vi "layout.vi"(0 "reference":refnum<class "FinalStateNode.lvclass">, 1 "graph":refnum<class "Graph.lvclass">, 2 "graphics":refnum<class "Graphics.lvclass">, 3 "grid":refnum<class "Grid.lvclass">, 5 "error in (no error)":errorcluster) -> (14 "reference out":refnum<class "FinalStateNode.lvclass">, 19 "error out":errorcluster)   [LabVIEW 2012, in "FinalStateNode.lvclass"]
doc: "public void layout(Graph g, Graphics2D g2, Grid grid)"
uses:
  <resource>/Framework/Providers/Open_GDS/UML/FinalStateNode_class/FinalStateNode.lvclass
  <resource>/Framework/Providers/Open_GDS/UML/Graph_class/Graph.lvclass
  <resource>/Framework/Providers/Open_GDS/UML/Graphics_class/Graphics.lvclass
  <resource>/Framework/Providers/Open_GDS/UML/Grid_class/Grid.lvclass
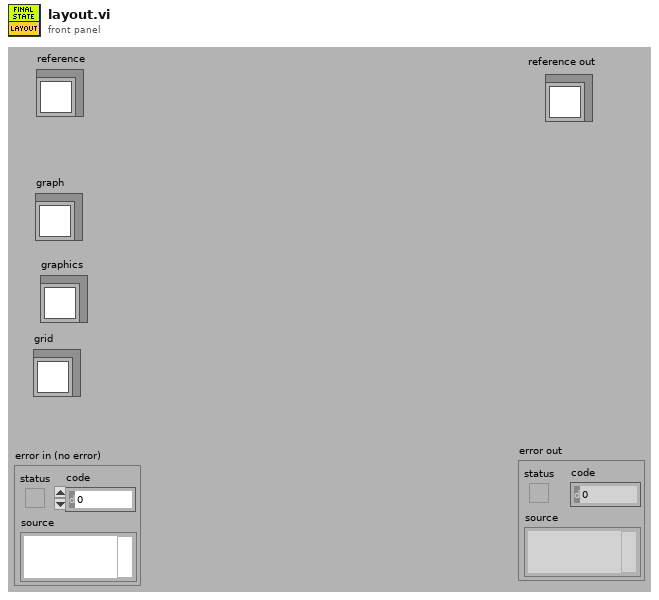
[diagram p1: front panel]
types:
  T1 = typedef "FinalStateNode.lvclass/ObjectAttributes.ctl" = cluster{"Base class":T2, "name":refnum<class "MultiLineString.lvclass">, "DEFAULT_WIDTH":i32, "DEFAULT_HEIGHT":i32}
  T2 = typedef "RectangularNode.lvclass/ObjectAttributes.ctl" = cluster{"Base class":T3, "bounds":T4}
  T3 = typedef "AbstractNode.lvclass/ObjectAttributes.ctl" = cluster{"parent":refnum<class "AbstractNode.lvclass">, "children":refnum<class "AbstractNode.lvclass">[], "Hidden":bool}
  T4 = typedef "Rectangle Rectangle2D.ctl" = cluster{"x":dbl, "y":dbl, "width":dbl, "height":dbl}
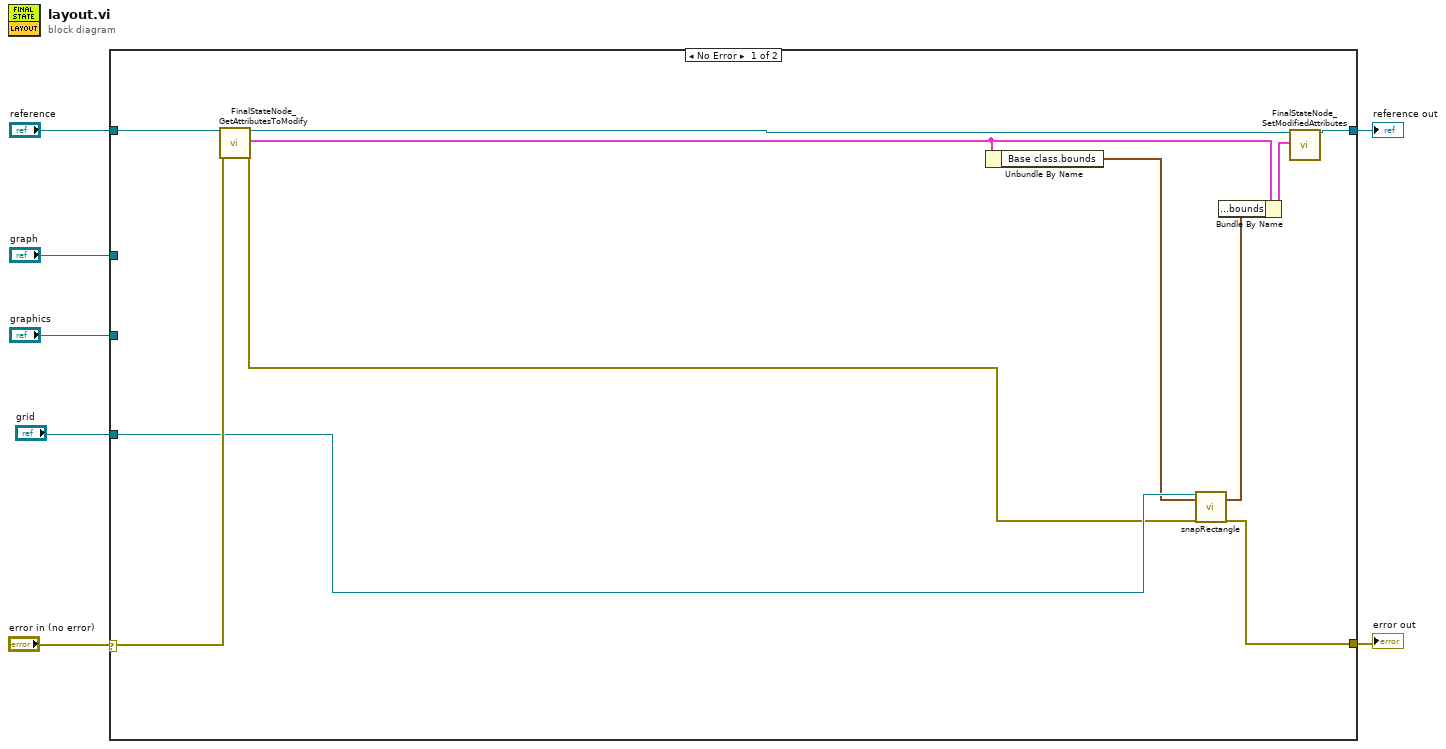
[diagram p0: block diagram]
diagram:
  n1 = case shown="No Error" "error in (no error)" {
    selector: "error in (no error)" -> [w15 w19]
    tunnel: "reference" -> [w18 w20]
    tunnel: [w17 w19] -> w6
    tunnel: [w16 w20] -> w5
    tunnel: "graph" -> [_ _]
    tunnel: "graphics" -> [_ _]
    tunnel: "grid" -> [w14 _]
    frame No Error {
      n2 = call <resource>:"FinalStateNode_GetAttributesToModify.vi"("reference in"=w18, "error in (no error)"=w15) -> ("reference out"=w11:refnum<class "FinalStateNode.lvclass">, "Attributes"=w13:T1, "error out"=w8:errorcluster)  [unwired: 1 in, 14 out]
      n3 = Unbundle By Name(w13) -> ("Base class.bounds"=w9:T4)
      n4 = call <resource>:"snapRectangle.vi"("reference"=w14, "bounds"=w9, "error in (no error)"=w8) -> ("boundsOut"=w12:T4, "error out"=w17:errorcluster)  [unwired: 15 out]
      n5 = Bundle By Name(cluster=w13, "Base class.bounds"=w12) -> (w10:T1)
      n6 = call <resource>:"FinalStateNode_SetModifiedAttributes.vi"("reference in"=w11, "Attributes"=w10) -> ("reference out"=w16:refnum<class "FinalStateNode.lvclass">)  [unwired: 4 in, 13 out]
    }
    frame Error {
    }
  }
  "reference out" <- w5
  "error out" <- w6
